vi "UIHandlerMain.vi"(6 "timeout_ms":i32=100, 8 "error in":errorcluster, 11 "UI_Manager in":refnum<class "UI_Library.lvclass">) -> (0 "error out":errorcluster, 3 "UI_Manager out":refnum<class "UI_Library.lvclass">, 4 "CloseUILoop":bool, 5 "#el_queue":i32)   [LabVIEW 2025, in "UI_Library.lvlib" / "UI_Library.lvclass"]
doc: "Update UI in accordance to the message received"
uses:
  UI_Library.lvclass
  UI_Library.lvclass/UI_Library.ctl
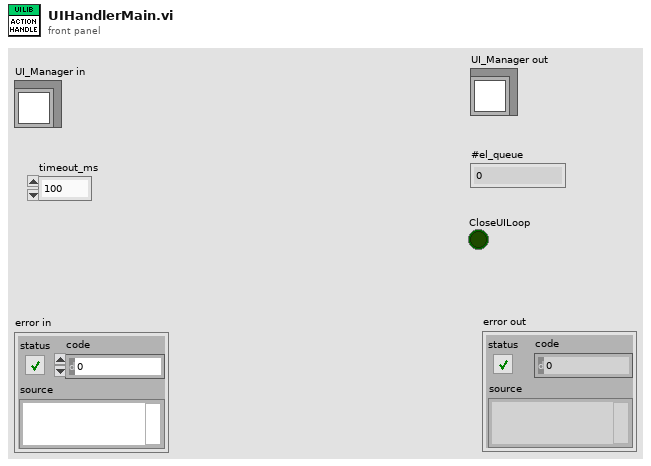
[diagram p1: front panel]
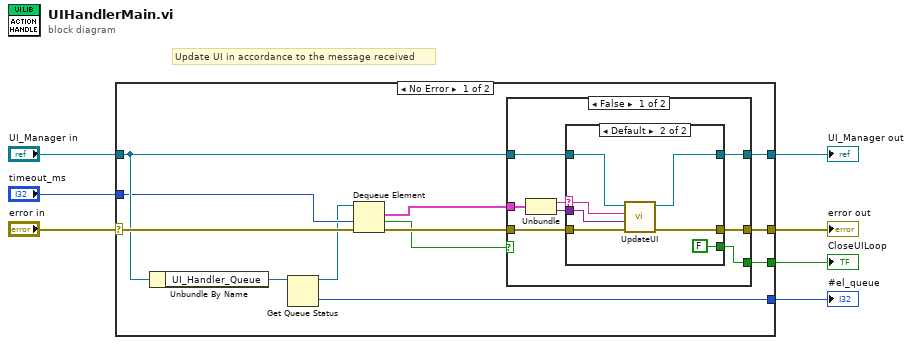
[diagram p0: block diagram]
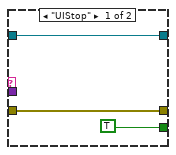
[diagram p2: hidden frame]
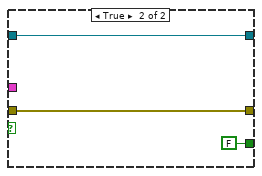
[diagram p3: hidden frame]
diagram:
  # "Update UI in accordance to the message received"
  n1 = case shown="No Error" "error in" {
    selector: "error in" -> [w19 w41]
    tunnel: "UI_Manager in" -> [w18 w42]
    tunnel: [w17 w42] -> w5
    tunnel: [w16 w41] -> w4
    tunnel: "timeout_ms" -> [w15 _]
    tunnel: [w14 _] -> w2
    tunnel: [w8 _] -> w1
    frame No Error {
      n2 = Unbundle By Name(w18) -> ("UI_Handler_Queue"=w13:refnum<queue>)
      n3 = Get Queue Status(queue=w13) -> (queue out=w9:refnum<queue>, # elements in queue=w14:i32)  [unwired: 2 in, 6 out]
      n4 = Dequeue Element(queue=w9, timeout in ms (-1)=w15, error in (no error)=w19) -> (element=w12:cluster{"cmd":string, "data":variant}, timed out?=w10:bool, error out=w11:errorcluster)  [unwired: 1 out]
      n5 = case shown="False" w10 {
        tunnel: w12 -> [w27 _]
        tunnel: w11 -> [w24 w39]
        tunnel: w18 -> [w23 w40]
        tunnel: [w22 w40] -> w17
        tunnel: [w21 w39] -> w16
        tunnel: [w20 FALSE] -> w8
        frame False {
          n6 = Unbundle(w27) -> ("cmd"=w26:string, "data"=w25:variant)
          n7 = case shown="Default" w26 {
            selector: w26 -> [_ w37]
            tunnel: w25 -> [_ w36]
            tunnel: w24 -> [w30 w35]
            tunnel: w23 -> [w29 w34]
            tunnel: [w29 w33] -> w22
            tunnel: [w30 w32] -> w21
            tunnel: [TRUE FALSE] -> w20
            frame "UIStop" {
            }
            frame Default {
              n8 = call-dynamic "UpdateUI.vi"("error in"=w35, "Control Data"=w36, "Action"=w37, "UI_Manager in"=w34) -> ("error out"=w32:errorcluster, "UI_Manager out"=w33:refnum<class "UI_Library.lvclass">)  [unwired: 6 in]
            }
          }
        }
        frame True {
        }
      }
    }
    frame Error {
    }
  }
  "UI_Manager out" <- w5
  "error out" <- w4
  "#el_queue" <- w2
  "CloseUILoop" <- w1
